vi "swerveTele.vi"(0 "joystickRight(x,y)":cluster{"X":dbl, "Y":dbl}, 1 "rotation":dbl, 3 "joystickLeft(x,y)":cluster{"X":dbl, "Y":dbl}, 4 "feildCentric":bool) -> (2 "drivePower":dbl[](array[numeric]), 5 "steerPower":dbl[](array[numeric]))   [LabVIEW 2019]
uses:
  swerveData.vi
  swerveOther/Theta Hypotenuse.vi
  swerveOther/Scale Power.vi
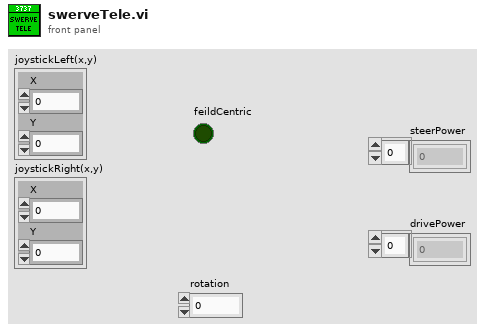
[diagram p1: front panel]
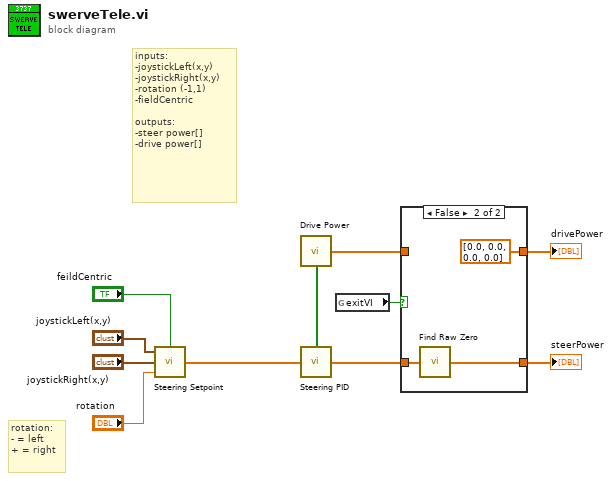
[diagram p0: block diagram]
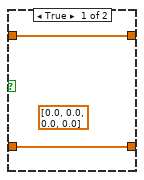
[diagram p2: hidden frame]
diagram:
  # "rotation:\n- = left\n+ = right"
  # "inputs:\n-joystickLeft(x,y)\n-joystickRight(x,y)\n-rotation (-1,1)\n-fieldCentric\n\noutputs:\n-steer power[]\n-drive power[]"
  n1 = call "Steering Setpoint.vi"("feildCentric"="feildCentric", "rotation"="rotation", "joystickRight(x,y)"="joystickRight(x,y)", "joystickLeft(x,y)"="joystickLeft(x,y)") -> ("steerSetpoint"=w9:dbl[])
  n2 = call "Steering PID.vi"("steeringSetpoints"=w9) -> ("invertPower"=w4:bool[], "steeringPower"=w8:dbl[])
  n3 = call "Drive Power.vi"("invertPower"=w4) -> ("drivePower"=w2:dbl[])  [unwired: 4 in]
  n4 = global read "swerveData.vi" "exitVI"() -> (w1:bool)
  n5 = case shown="False" w1 {
    tunnel: w8 -> [w12 w16]
    tunnel: [w12 w15] -> w7
    tunnel: [w13 dbl[] [0.0, 0.0, 0.0, 0.0] ("drivePower")] -> w3
    tunnel: w2 -> [w13 _]
    frame True {
      (unwired) dbl[] [0.0, 0.0, 0.0, 0.0] ("drivePower")
    }
    frame False {
      n6 = call "Find Raw Zero.vi"("steeringPower"=w16) -> ("powerOutput"=w15:dbl[])
    }
  }
  "steerPower" <- w7
  "drivePower" <- w3
